vi "set_DataCollection_specification.vi"(8 "error in (no error)":errorcluster, 9 "DataCollection adapter path":string, 10 "DataCollection specification":T1, 11 "ScanModeDL090923Scaffold in":refnum<class "ImagingModeDL090923Scaffold.lvclass">) -> (0 "error out":errorcluster, 3 "ScanModeDL090923Scaffold out":refnum<class "ImagingModeDL090923Scaffold.lvclass">)   [LabVIEW 2010, in "ImagingModeDL090923Scaffold.lvclass"]
uses:
  ImagingModeDL090923Scaffold.lvclass
  common/clusters/plugin_specification.ctl
  ImagingModeDL090923Scaffold.lvclass/ImagingModeDL090923Scaffold.ctl
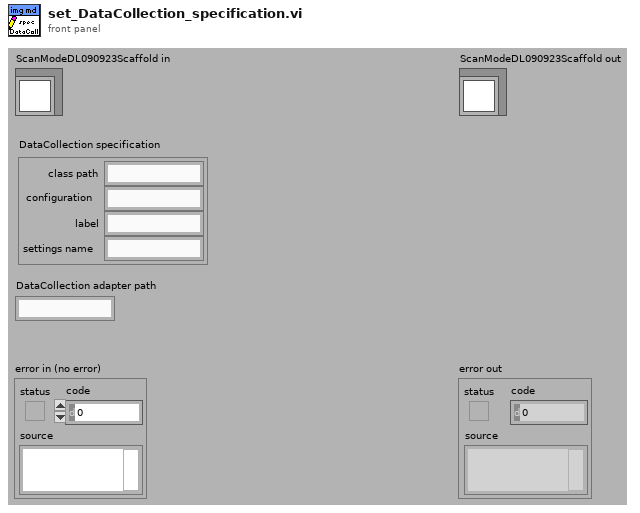
[diagram p1: front panel]
types:
  T1 = typedef "plugin_specification.ctl" = cluster{"class path":string, "configuration":string, "label":string, "settings name":string}
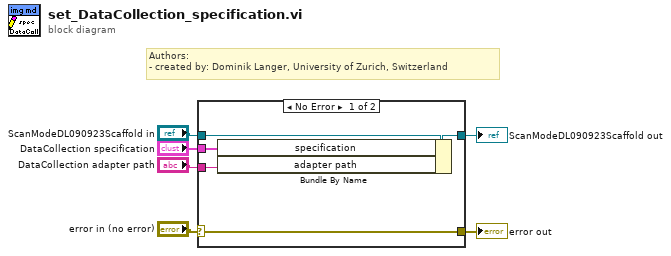
[diagram p0: block diagram]
diagram:
  # "Authors: \n- created by: Dominik Langer, University of Zurich, Switzerland"
  n1 = case shown="No Error" "error in (no error)" {
    selector: "error in (no error)" -> [w11 w12]
    tunnel: [w11 w12] -> w5
    tunnel: [w9 w13] -> w3
    tunnel: "ScanModeDL090923Scaffold in" -> [w10 w13]
    tunnel: "DataCollection specification" -> [w8 _]
    tunnel: "DataCollection adapter path" -> [w7 _]
    frame No Error {
      n2 = Bundle By Name(cluster=w10, "specification"=w8, "adapter path"=w7) -> (w9:refnum<class "ImagingModeDL090923Scaffold.lvclass">)
    }
    frame Error {
    }
  }
  "error out" <- w5
  "ScanModeDL090923Scaffold out" <- w3
